vi "SC10_set_trigger_mode.vi"() -> ()   [LabVIEW 2010]
panel:
  in  "trigger mode":i32(ring) items=["internal", "external"]
  out "substring":string
  in  "VISA resource name":refnum<visa-resource-name>
  out "VISA resource name out":refnum<visa-resource-name>
  out "read buffer":string
  out "return count 2":u32
  out "return count":u32
  out "error out":errorcluster
  in  "error in (no error)":errorcluster
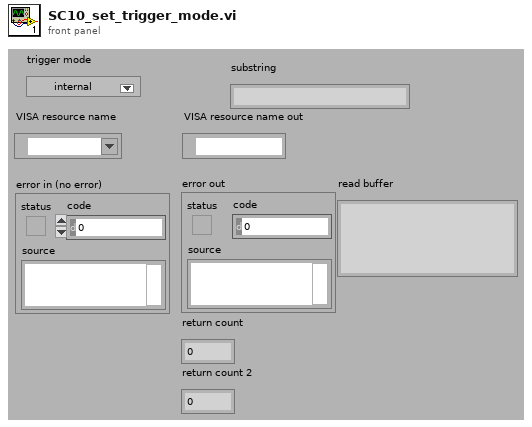
[diagram p1: front panel]
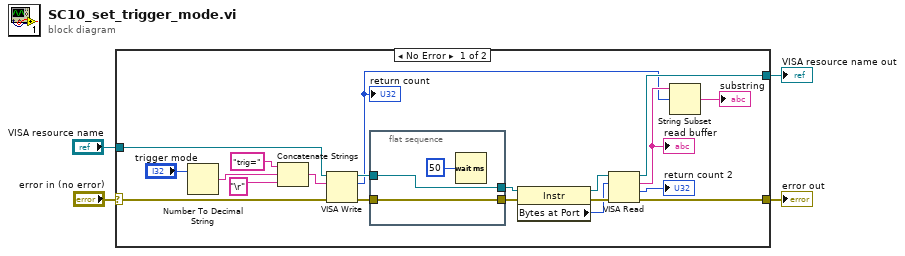
[diagram p0: block diagram]
diagram:
  n1 = case shown="No Error" "error in (no error)" {
    selector: "error in (no error)" -> [w22 w28]
    tunnel: [w21 w28] -> w3
    tunnel: [w19 w29] -> w2
    tunnel: "VISA resource name" -> [w18 w29]
    frame No Error {
      n2 = Number To Decimal String(number="trigger mode") -> (decimal integer string=w12:string)  [unwired: 1 in]
      n3 = Concatenate Strings("trig=" ("write buffer"), w12, "\r" ("string")) -> (w11:string)
      n4 = VISA Write(VISA resource name=w18, write buffer=w11, error in (no error)=w22) -> (VISA resource name out=w24:refnum<visa-resource-name>, return count=w15:u32, error out=w23:errorcluster)
      "return count" <- w15
      n5 = flat-sequence {
        tunnel: w24 -> [w26]
        tunnel: [w26] -> w7
        tunnel: w23 -> [w25]
        tunnel: [w25] -> w6
        frame #0 {
          n6 = Wait (ms)(milliseconds to wait=u32 50) -> ()  [unwired: 1 out]
        }
      }
      n7 = property class="Instr"(reference=w7, error in=w6) -> (reference out=w8:refnum<visa-resource-name>, error out=w9:errorcluster, "Bytes at Port"=w5:u32)
      n8 = VISA Read(VISA resource name=w8, byte count=w5, error in (no error)=w9) -> (VISA resource name out=w19:refnum<visa-resource-name>, read buffer=w17:string, return count=→"return count 2":u32, error out=w21:errorcluster)
      "read buffer" <- w17
      n9 = String Subset(string=w17, offset (0)=w15) -> (substring=→"substring":string)  [unwired: 1 in]
    }
    frame Error {
    }
  }
  "error out" <- w3
  "VISA resource name out" <- w2
